vi "Set Color To Caller.vi"(8 "error in (no error)":errorcluster, 11 "Setting View in":refnum<class "Setting View.lvclass">) -> (0 "error out":errorcluster, 3 "Setting View out":refnum<class "Setting View.lvclass">)   [LabVIEW 2020, in "[V]Setting View.lvlib" / "Setting View.lvclass"]
uses:
  Setting View.lvclass
  C:/Program Files (x86)/National Instruments/LabVIEW 2020/vi.lib/ActorFramework/Actor/Actor.lvclass
  <vilib>/ActorFramework/Message/Message.lvclass
  Setting View.lvclass/Setting View.ctl
  Depden On/MVVM Framework/MVVM Abstruct View/MVVM Abstruct View/MVVM Abstruct View.lvclass/MVVM Abstruct View.ctl
  <vilib>/ActorFramework/Actor/Actor.lvclass/Actor.ctl
  <vilib>/ActorFramework/Message Enqueuer/Message Enqueuer.lvclass/Message Enqueuer.ctl
  Color Interface/Color Interface Messages/Set Color Msg/Set Color Msg.lvclass/Set Color Msg.ctl
  Depden On/MVVM Framework/MVVM Abstruct View/MVVM Abstruct View/Accessor/Read ActorMap-Views.vi
  <vilib>/ActorFramework/Message Enqueuer/Init from Existing Queue.vi
  Color Interface/Color Interface Messages/Set Color Msg/Set Color Msg.lvclass
  C:/Program Files (x86)/National Instruments/LabVIEW 2020/vi.lib/ActorFramework/Message/Message.lvclass
  <vilib>/ActorFramework/Stop Msg/Stop Msg.lvclass
  <vilib>/ActorFramework/Message Priority Queue/Priority Enqueue.vi
  Depden On/ActorMap/ActorMap.lvclass
  <vilib>/ActorFramework/Message Enqueuer/Message Enqueuer.lvclass
  <vilib>/ActorFramework/Actor/Actor.lvclass
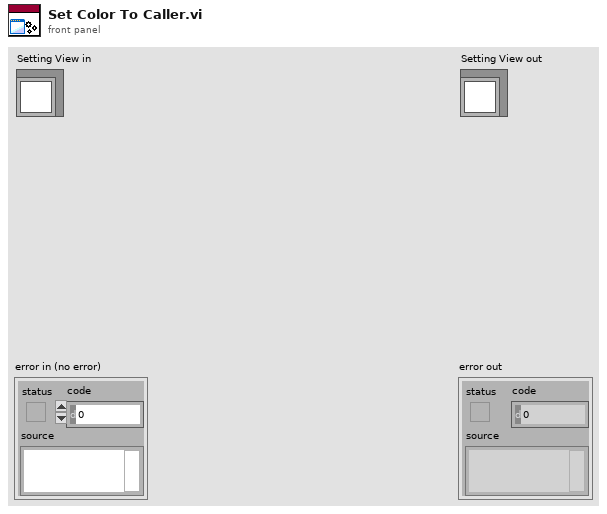
[diagram p1: front panel]
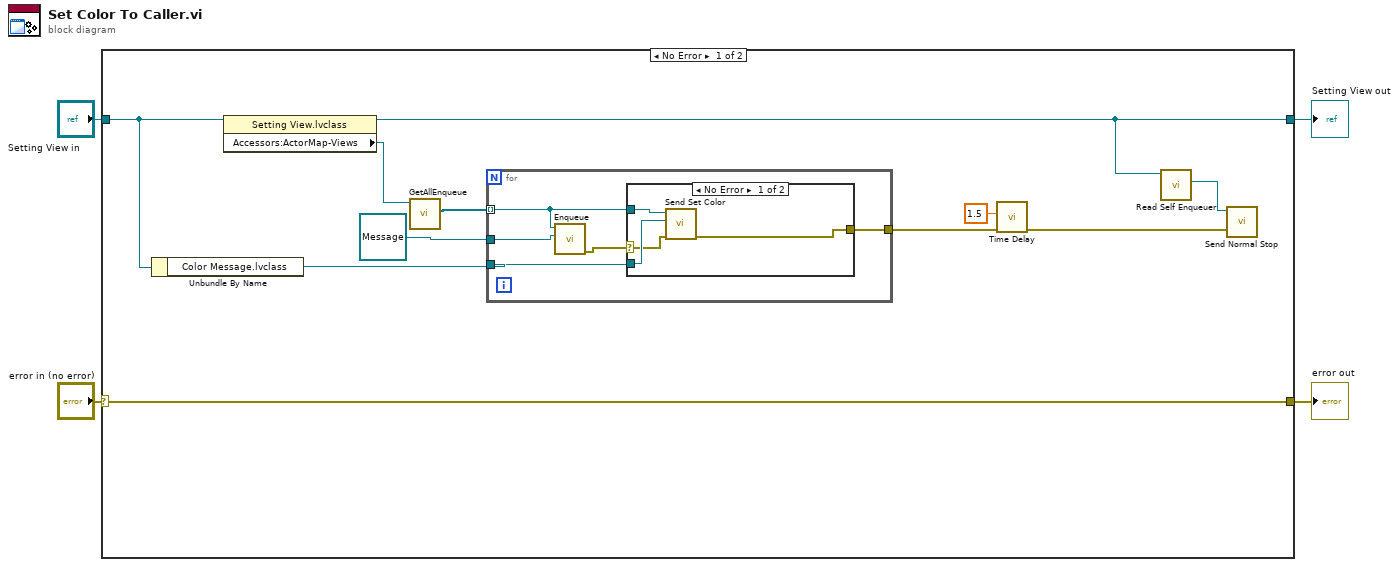
[diagram p0: block diagram]
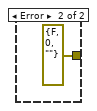
[diagram p2: hidden frame]
diagram:
  n1 = case shown="No Error" "error in (no error)" {
    selector: "error in (no error)" -> [w15 w27]
    tunnel: [w15 w27] -> w3
    tunnel: [w12 w26] -> w1
    tunnel: "Setting View in" -> [w8 w26]
    frame No Error {
      n2 = Unbundle By Name(w8) -> ("Color Message.lvclass"=w7:refnum<class "Color Message.lvclass">)
      n3 = property class="Setting View.lvclass"(reference=w8) -> (reference out=w12:refnum<class "Setting View.lvclass">, "Accessors:ActorMap-Views"=w10:refnum<class "ActorMap.lvclass">)  [unwired: 1 in, 1 out]
      n4 = call "GetAllEnqueue.vi"("ActorMap in"=w10) -> ("Enqueues"=w9:refnum<class "Message Enqueuer.lvclass">[])  [unwired: 7 in, 3 out]
      n5 = for {
        tunnel: [w20] -> w11
        tunnel: w9 -> [w18] mode=indexing
        tunnel: w7 -> [w19]
        tunnel: refnum<class "Message.lvclass"> refnum ("Message") -> [w17]
        n6 = call <vilib>:"Enqueue.vi"("Message"=w17, "Message Enqueuer in"=w18) -> ("error out"=w16:errorcluster)  [unwired: 8 in, 1 out]
        n7 = case shown="No Error" w16 {
          selector: w16 -> [w21 _]
          tunnel: [w24 errorcluster {"status"=FALSE, "code"=0, "source"=""} ("error out")] -> w20
          tunnel: w19 -> [w23 _]
          tunnel: w18 -> [w22 _]
          frame No Error {
            n8 = call "Send Set Color.vi"("error in (no error)"=w21, "Color Message.lvclass"=w23, "Message Enqueuer"=w22) -> ("error out"=w24:errorcluster)  [unwired: 7 in, 1 out]
          }
          frame Error {
          }
        }
      }
      n9 = call "Time Delay"("error in (no error)"=w11, "Delay Time (s)"=1.5) -> ("error out"=w14:errorcluster)  [unwired: 9 in]
      n10 = call <vilib>:"Read Self Enqueuer.vi"("Actor"=w12) -> ("Self Enqueuer"=w13:refnum<class "Message Enqueuer.lvclass">)  [unwired: 10 in]
      n11 = call <vilib>:"Send Normal Stop.vi"("error in (no error)"=w14, "Message Enqueuer"=w13) -> ()  [unwired: 9 in, 1 out]
    }
    frame Error {
    }
  }
  "error out" <- w3
  "Setting View out" <- w1
